vi "DriveDistanceSubVi.vi"(4 "navX Device":T5 {"Interface"."Update Rate (4Hz-60Hz)" min=4 max=60 step=1}, 5 "EncoderDevRefLeft":T1, 6 "EncoderDevRefRight":T1, 7 "Setpoint":dbl, 8 "Angle":dbl, 9 "Deadband":dbl, 10 "VDeadband":dbl, 11 "Speed":dbl) -> (3 "Boolean":bool)   [LabVIEW 2015]
uses:
  NavX/navX Library v2/TypeDefs/Z900_navX_DeviceTypeDef.ctl
  NavX/navX Library v2/TypeDefs/Z900_navX_ProtocolTypeDef.ctl
  NavX/navX Library v2/TypeDefs/Z900_navX_NotifyPacketTypeDef.ctl
  NavX/navX Library v2/TypeDefs/Z900_navX_ActionTypeDef.ctl
  <vilib>/Rock Robotics/WPI/Encoder/WPI_EncoderDevRef.ctl
  <vilib>/Rock Robotics/SystemInterfaces/Encoder/FPGA_EncoderIdx.ctl
  <vilib>/Rock Robotics/SystemInterfaces/Counter/FPGA_CounterCtrSystemIndex.ctl
  <vilib>/Rock Robotics/WPI/Encoder/WPI_EncoderType.ctl
  <vilib>/Rock Robotics/Network Tables/NT Read Number.vi
  <vilib>/addons/control/pid/pid.llb/PID (DBL).vi
  <vilib>/addons/control/pid/NI_PID_pid.lvlib
  NavX/navX Library v2/navX Library v2.lvlib
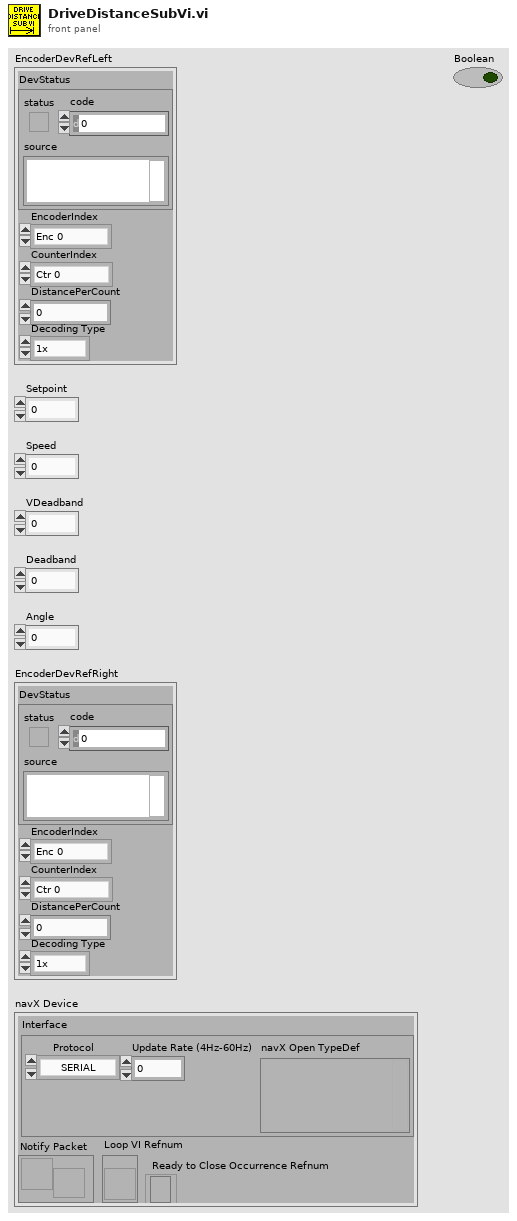
[diagram p1: front panel]
types:
  T1 = typedef "WPI_EncoderDevRef.ctl" = cluster{"DevStatus":errorcluster, "EncoderIndex":T2, "CounterIndex":T3, "DistancePerCount":dbl, "Decoding Type":T4}
  T2 = typedef "FPGA_EncoderIdx.ctl" = enum8{"Enc 0", "Enc 1", "Enc 2", "Enc 3", "Enc 4", "Enc 5", "Enc 6", "Enc 7", "Invalid"}
  T3 = typedef "FPGA_CounterCtrSystemIndex.ctl" = enum8{"Ctr 0", "Ctr 1", "Ctr 2", "Ctr 3", "Ctr 4", "Ctr 5", "Ctr 6", "Ctr 7", "Invalid"}
  T4 = typedef "WPI_EncoderType.ctl" = enum16{"1x", "2x", "4x"}
  T5 = typedef "navX Library v2.lvlib/Z900_navX_DeviceTypeDef.ctl" = cluster{"Interface":cluster{"Protocol":T6, "Update Rate (4Hz-60Hz)":u8, "navX Open TypeDef":variant}, "Notify Packet":refnum<notifier>, "Loop VI Refnum":refnum<vi>, "Ready to Close Occurrence Refnum":refnum<k4>}
  T6 = typedef "navX Library v2.lvlib/Z900_navX_ProtocolTypeDef.ctl" = enum16{"SERIAL", "I2C", "SPI"}
  T7 = cluster{"Numeric":dbl, "Numeric":dbl, "Numeric":dbl}
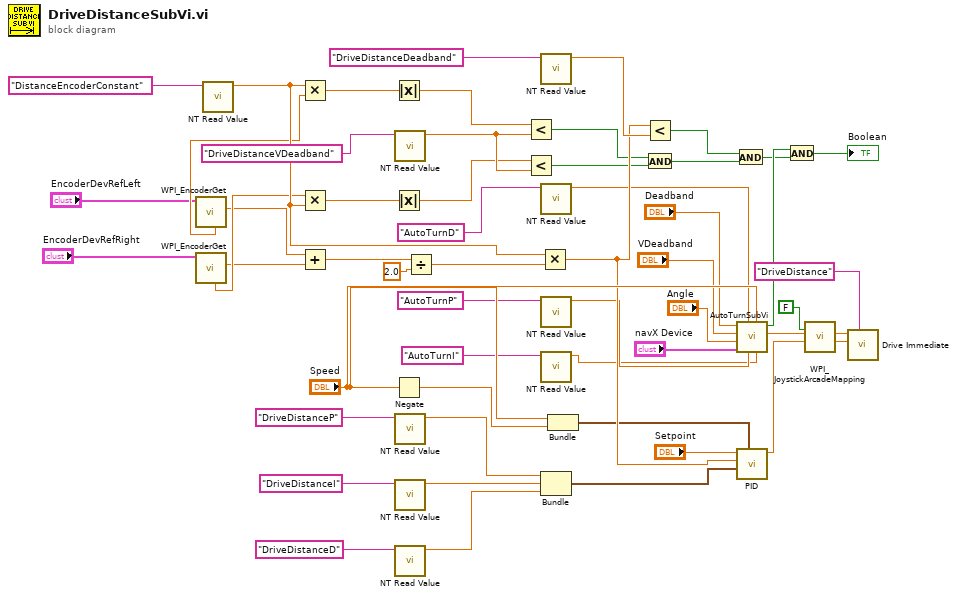
[diagram p0: block diagram]
diagram:
  n1 = call <vilib>:"WPI_EncoderGet.vi"("EncoderDevRef"="EncoderDevRefLeft") -> ("Distance"=w5:dbl, "Rate"=w40:dbl)  [unwired: 5 in, 4 out]
  n2 = call <vilib>:"WPI_EncoderGet.vi"("EncoderDevRef"="EncoderDevRefRight") -> ("Distance"=w6:dbl, "Rate"=w38:dbl)  [unwired: 5 in, 4 out]
  n3 = call-poly <vilib>:"NT Read Value.vi"("Name"="DistanceEncoderConstant") -> ("Numeric"=w41:dbl)  [unwired: 9 in, 1 out]
  n4 = Multiply(x=w41, y=w40) -> (x*y=w39:dbl)
  n5 = Multiply(x=w38, y=w41) -> (x*y=w37:dbl)
  n6 = Add(x=w5, y=w6) -> (x+y=w7:dbl)
  n7 = Absolute Value(x=w39) -> (abs(x)=w47:dbl)
  n8 = Absolute Value(x=w37) -> (abs(x)=w46:dbl)
  n9 = Negate(x="Speed") -> (-x=w11:dbl)
  n10 = call-poly <vilib>:"NT Read Value.vi"("Name"="DriveDistanceVDeadband") -> ("Numeric"=w48:dbl)  [unwired: 9 in, 1 out]
  n11 = call-poly <vilib>:"NT Read Value.vi"("Name"="DriveDistanceP") -> ("Numeric"=w29:dbl)  [unwired: 9 in, 1 out]
  n12 = call-poly <vilib>:"NT Read Value.vi"("Name"="DriveDistanceI") -> ("Numeric"=w28:dbl)  [unwired: 9 in, 1 out]
  n13 = call-poly <vilib>:"NT Read Value.vi"("Name"="DriveDistanceD") -> ("Numeric"=w27:dbl)  [unwired: 9 in, 1 out]
  n14 = Divide(x=w7, y=2.0) -> (x/y=w9:dbl)
  n15 = Less?(x=w47, y=w48) -> (x < y?=w35:bool)
  n16 = Less?(x=w46, y=w48) -> (x < y?=w36:bool)
  n17 = Multiply(x=w41, y=w9) -> (x*y=w42:dbl)
  n18 = call-poly <vilib>:"NT Read Value.vi"("Name"="DriveDistanceDeadband") -> ("Numeric"=w43:dbl)  [unwired: 9 in, 1 out]
  n19 = call-poly <vilib>:"NT Read Value.vi"("Name"="AutoTurnD") -> ("Numeric"=w21:dbl)  [unwired: 9 in, 1 out]
  n20 = call-poly <vilib>:"NT Read Value.vi"("Name"="AutoTurnP") -> ("Numeric"=w23:dbl)  [unwired: 9 in, 1 out]
  n21 = call-poly <vilib>:"NT Read Value.vi"("Name"="AutoTurnI") -> ("Numeric"=w22:dbl)  [unwired: 9 in, 1 out]
  n22 = Bundle("Numeric"=w29, "Numeric"=w28, "Numeric"=w27) -> (w13:T7)  [unwired: 1 in]
  n23 = Bundle("Speed"="Speed", w11) -> (w12:cluster{"Speed":dbl, dbl})  [unwired: 1 in]
  n24 = Less?(x=w42, y=w43) -> (x < y?=w45:bool)
  n25 = And(x=w35, y=w36) -> (x .and. y?=w44:bool)
  n26 = And(x=w45, y=w44) -> (x .and. y?=w52:bool)
  n27 = call "AutoTurnSubVi.vi"("I"=w22, "Speed"="Speed", "P"=w23, "D"=w21, "navX Device"="navX Device", "Angle"="Angle", "VDeadband"="VDeadband", "Deadband"="Deadband") -> ("Output"=w49:dbl, "Boolean"=w53:bool)  [unwired: 2 in]
  n28 = call-poly <vilib>:"PID.vi"("output range"=w12, "PID gains"=w13, "process variable"=w42, "setpoint"="Setpoint") -> ("output"=w50:dbl)  [unwired: 6 in, 1 out]
  n29 = And(x=w53, y=w52) -> (x .and. y?=→"Boolean":bool)
  n30 = call <vilib>:"WPI_JoystickArcadeMapping.vi"("Square Inputs"=FALSE, "Y axis value"=w50, "X axis value"=w49) -> ("Right Motor Value"=w15:dbl, "Left Motor Value"=w14:dbl)  [unwired: 7 in]
  n31 = call "Drive Immediate.vi"("Description"="DriveDistance", "Right Setpoint"=w15, "Left Setpoint"=w14) -> ()  [unwired: 8 in, 1 out]
